vi "_macro_Choreo_GetDifferentialTrajectory.vi"() -> ()   [LabVIEW 2019, in "ChoreoLib.lvlib"]
uses:
  ChoreoLib.lvlib
  TypeDef/ChoreoTrajectoryDifferential.ctl
  TypeDef/ChoreoDifferentialSample.ctl
  TypeDef/ChoreoEventMarker.ctl
panel:
  out "ChoreoTrajectoryDifferential":T1
  out "error out":errorcluster
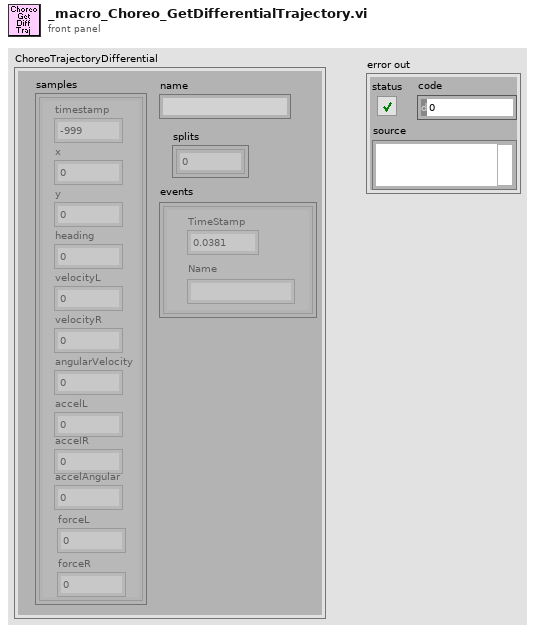
[diagram p1: front panel]
types:
  T1 = typedef "ChoreoLib.lvlib/ChoreoTrajectoryDifferential.ctl" = cluster{"name":string, "samples":T2[], "splits":i32[], "events":T3[]}
  T2 = typedef "ChoreoLib.lvlib/ChoreoDifferentialSample.ctl" = cluster{"timestamp":dbl, "x":dbl, "y":dbl, "heading":dbl, "velocityL":dbl, "velocityR":dbl, "angularVelocity":dbl, "accelL":dbl, "accelR":dbl, "accelAngular":dbl, "forceL":dbl, "forceR":dbl}
  T3 = typedef "ChoreoLib.lvlib/ChoreoEventMarker.ctl" = cluster{"TimeStamp":dbl, "Name":string}
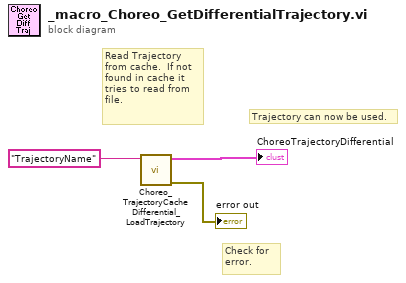
[diagram p0: block diagram]
diagram:
  # "Trajectory can now be used."
  # "Check for \nerror."
  # "Read Trajectory\nfrom cache.  If not\nfound in cache it\ntries to read from\nfile."
  n1 = call "Choreo_TrajectoryCacheDifferential_LoadTrajectory.vi"("TrajectoryName"="TrajectoryName" ("FileName")) -> ("error out"=→"error out":errorcluster, "ChoreoTrajectoryDifferential"=→"ChoreoTrajectoryDifferential":T1)  [unwired: 9 in]
